vi "HUD.vi"() -> ()   [LabVIEW 2019]
uses:
  <vilib>/Rock Robotics/WPI/DriverStation/WPI_DriverStationAllianceInfo.ctl
panel:
  in  "Alliance":T1
  in  "Control panel done":bool
  in  "Control panel up":bool
  in  "Elevator Up":bool
  in  "Intake Out":bool
  in  "Shooter aligned":bool
  in  "Shooter up":bool
  in  "Balls in":bool
  out "Image":T2(plugin-control)
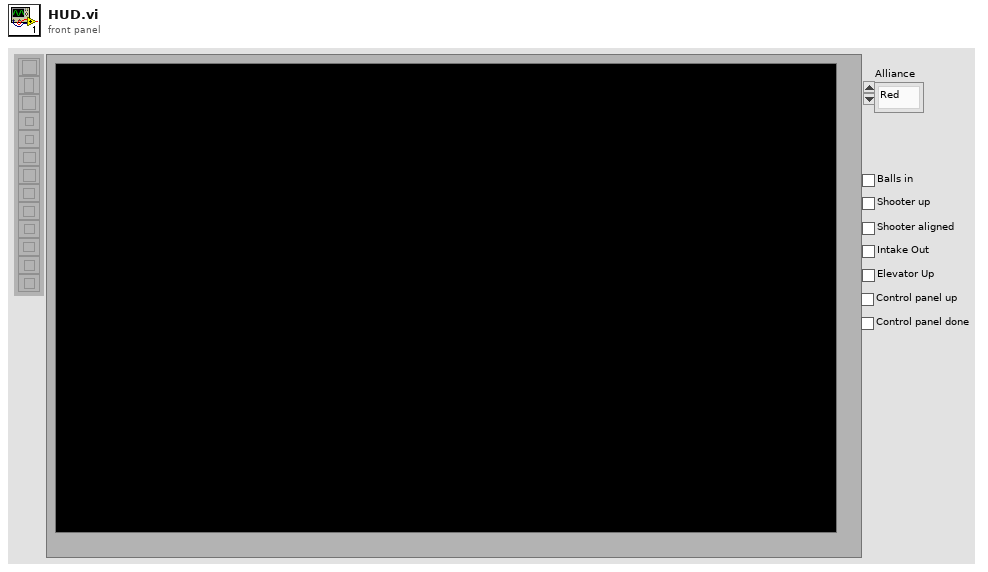
[diagram p1: front panel]
types:
  T1 = typedef "WPI_DriverStationAllianceInfo.ctl" = enum16{"Red", "Blue", "Invalid"}
  T2 = typedef "IMAQ Image.ctl" = refnum<image>
  T3 = typedef "Image Type" = u32
  T4 = enum32{"invalid app kind", "Development System", "Run Time System", "Student Edition", "Embedded LabVIEW", "Evaluation", "Custom"}
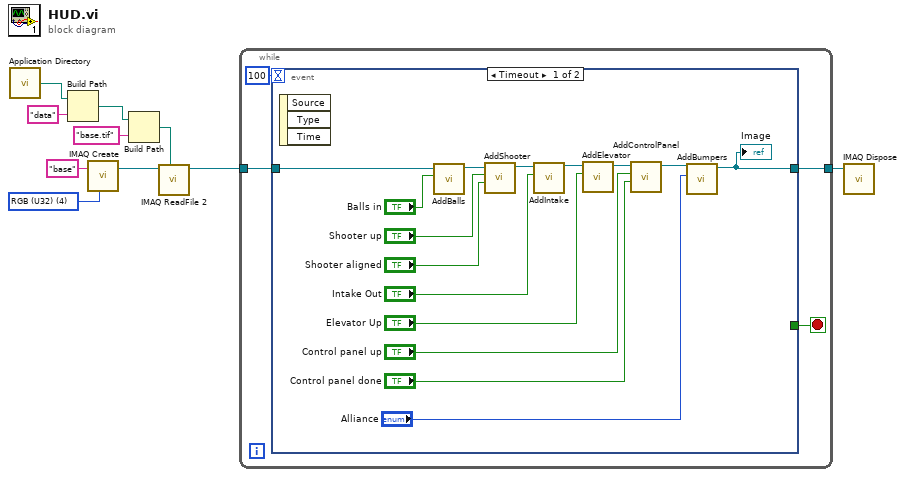
[diagram p0: block diagram]
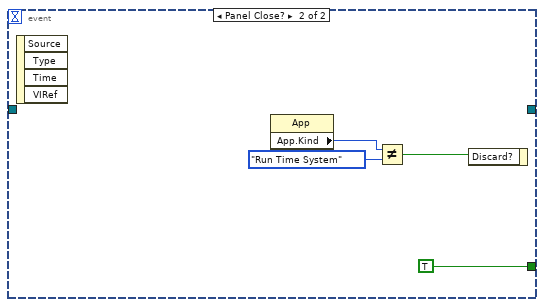
[diagram p2: hidden frame]
diagram:
  w9 = T3 4 items=["Grayscale (U8)", "Grayscale (I16)", "Grayscale (SGL)", "Complex (CSG)", "RGB (U32)", "HSL (U32)", "RGB (U64)", "Grayscale (U16)"] ("Image Type")
  n1 = call <vilib>:"Application Directory.vi"() -> ("Application Directory"=w3:path)
  n2 = Build Path(base path=w3, name or relative path="data") -> (appended path=w4:path)
  n3 = call "IMAQ Create"("Image Name"="base", "Image Type"=w9) -> ("New Image"=w8:T2)  [unwired: 3 in, 1 out]
  n4 = Build Path(base path=w4, name or relative path="base.tif") -> (appended path=w5:path)
  n5 = call "IMAQ ReadFile 2"("File Path"=w5, "Image"=w8) -> ("Image Out"=w6:T2)  [unwired: 5 in, 4 out]
  n6 = while {
    tunnel: w6 -> [w13]
    tunnel: [w12] -> w7
    stop <- w11 stop-if-true
    n7 = event shown="[0] Timeout" {
      selector: _ -> [_ _]
      dyn-events: _ -> [_ _]
      timeout: 100 -> [_ _]
      tunnel: w13 -> [w29 _]
      tunnel: [w16 _] -> w12
      tunnel: [_ TRUE] -> w11
      event Timeout {
        n8 = event-data() -> ()  [unwired: 1 in, 3 out]
        n9 = call "AddBalls.vi"("Balls in"="Balls in", "Refnum in"=w29) -> ("Refnum out"=w27:T2)  [unwired: 9 in]
        n10 = call "AddShooter.vi"("Shooter Aligned"="Shooter aligned", "Shooter Up"="Shooter up", "Refnum in"=w27) -> ("Refnum out"=w24:T2)  [unwired: 8 in]
        n11 = call "AddIntake.vi"("Intake out"="Intake Out", "Refnum in"=w24) -> ("Refnum out"=w20:T2)  [unwired: 9 in]
        n12 = call "AddElevator.vi"("Elevator Up"="Elevator Up", "Refnum in"=w20) -> ("Refnum out"=w19:T2)  [unwired: 9 in]
        n13 = call "AddControlPanel.vi"("Control panel done"="Control panel done", "Control panel up"="Control panel up", "Refnum in"=w19) -> ("Refnum out"=w17:T2)  [unwired: 8 in]
        n14 = call "AddBumpers.vi"("Alliance"="Alliance", "Refnum in"=w17) -> ("Refnum out"=w16:T2)  [unwired: 9 in]
        "Image" <- w16
      }
      event Panel Close? {
        n15 = event-data() -> ()  [unwired: 1 in, 4 out]
        n16 = property class="App"() -> ("App.Kind"=w32:T4)  [unwired: 2 in, 2 out]
        n17 = Not Equal?(x=w32, y=T4."Run Time System") -> (x != y?=w31:bool)
        n18 = event-data("Discard?"=w31) -> ()  [unwired: 1 in, 1 out]
      }
    }
  }
  n19 = call "IMAQ Dispose"("Image"=w7) -> ()  [unwired: 5 in, 1 out]
